vi "Launcher.vi"   [LabVIEW 2020, in "Test-MM.lvlib"]
uses:
  Test-MM.lvlib
  Test-MM/Test-MM.lvclass
  C:/Program Files (x86)/National Instruments/LabVIEW 2020/vi.lib/ActorFramework/Actor/Actor.lvclass
  <vilib>/ActorFramework/Actor/Actor.lvclass
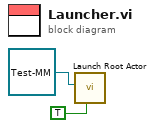
[diagram p0: block diagram]
diagram:
  n1 = call <vilib>:"Launch Root Actor.vi"("Open Actor Core front panel? (F)"=TRUE, "Actor"=refnum<class "Test-MM.lvclass"> refnum ("Test-MM.lvlib:Test-MM.lvclass")) -> ()  [unwired: 8 in, 2 out]
